vi "Self-Test.vi"(8 "error in (no error)":errorcluster, 11 "VISA resource name":refnum<visa-resource-name>) -> (0 "error out":errorcluster, 1 "Self-Test Result Message":string, 2 "Self-Test Result Code":i32, 3 "VISA resource name out":refnum<visa-resource-name>)   [LabVIEW 2015, in "LeCroy Wave Series.lvlib"]
doc: "This VI runs the instrument's self test routine and returns the test results."
uses:
  <instrlib>/LeCroy Wave Series/LeCroy Wave Series.lvlib
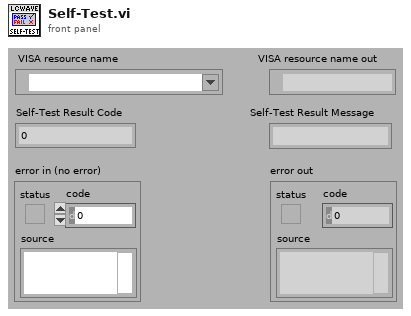
[diagram p1: front panel]
types:
  T1 = cluster{"Status":bool, "Code":i32, "Source (VI Name)":string}
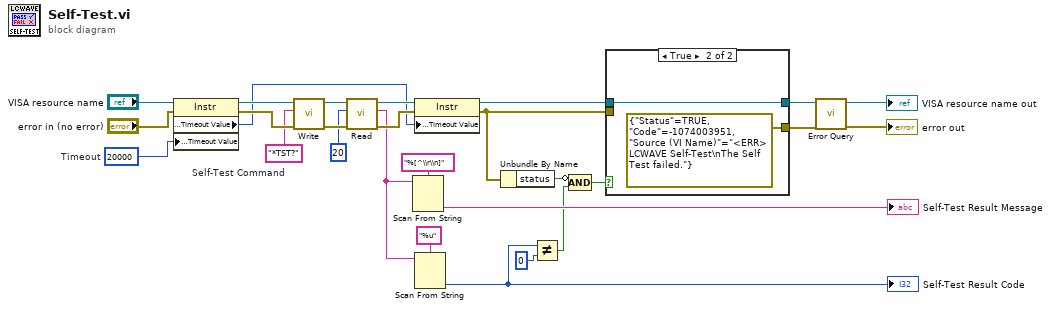
[diagram p0: block diagram]
diagram:
  w16 = u32 20000  # Timeout
  w12 = "*TST?"  # Self-Test Command
  n1 = property on="Property Node" class="Instr"(reference="VISA resource name", error in="error in (no error)", "General Settings:Timeout Value"=w16) -> (reference out=w14:refnum<visa-resource-name>, error out=w15:errorcluster, "General Settings:Timeout Value"=w13:u32)
  n2 = call <instrlib>:"Write.vi"("error in (no error)"=w15, "Write Buffer"=w12, "VISA resource name"=w14) -> ("error out"=w22:errorcluster, "VISA resource name out"=w23:refnum<visa-resource-name>)  [unwired: 6 in, 1 out]
  n3 = call <instrlib>:"Read.vi"("error in (no error)"=w22, "Byte Count"=u32 20 ("byte count (20)"), "VISA resource name"=w23) -> ("error out"=w24:errorcluster, "Read Buffer"=w18:string, "VISA resource name out"=w25:refnum<visa-resource-name>)  [unwired: 5 in, 1 out]
  n4 = Scan From String(format string="%[^\\r\\n]" ("Format String"), input string=w18) -> (output 1=→"Self-Test Result Message":string)  [unwired: 3 in, 3 out]
  n5 = property on="Property Node" class="Instr"(reference=w25, error in=w24, "General Settings:Timeout Value"=w13) -> (reference out=w11:refnum<visa-resource-name>, error out=w10:errorcluster)
  n6 = Scan From String(format string="%u", input string=w18) -> (output 1=w6:i32)  [unwired: 3 in, 3 out]
  "Self-Test Result Code" <- w6
  n7 = Unbundle By Name(w10) -> ("status"=w8:bool)
  n8 = Not Equal?(x=w6, y=0) -> (x != y?=w9:bool)
  n9 = Compound Arithmetic op=AND(invert w8, w9) -> (w7:bool)
  n10 = case shown="True" w7 {
    tunnel: w11 -> [w29 w31]
    tunnel: w10 -> [w28 _]
    tunnel: [w28 T1 {"Status"=TRUE, "Code"=-1074003951, "Source (VI Name)"="<ERR> LCWAVE Self-Test\nThe Self Test failed."}] -> w3
    tunnel: [w29 w31] -> w4
    frame False {
    }
    frame True {
    }
  }
  n11 = call <instrlib>:"Error Query.vi"("error in (no error)"=w3, "VISA resource name"=w4) -> ("error out"=→"error out":errorcluster, "VISA resource name out"=→"VISA resource name out":refnum<visa-resource-name>)  [unwired: 6 in, 2 out]
